vi "get_instrument_ID.vi"(8 "error in (no error)":errorcluster, 10 "ID Command":string="*IDN?\n", 11 "Function Generator in":refnum<class "Function Generator.lvclass">) -> (0 "error out":errorcluster, 2 "Instrument ID":string, 3 "Function Generator out":refnum<class "Function Generator.lvclass">)   [LabVIEW 2020, in "Function Generator.lvclass"]
uses:
  Function Generator.lvclass
  Function Generator.lvclass/Function Generator.ctl
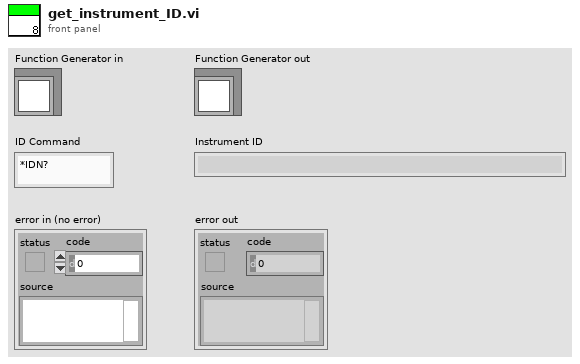
[diagram p1: front panel]
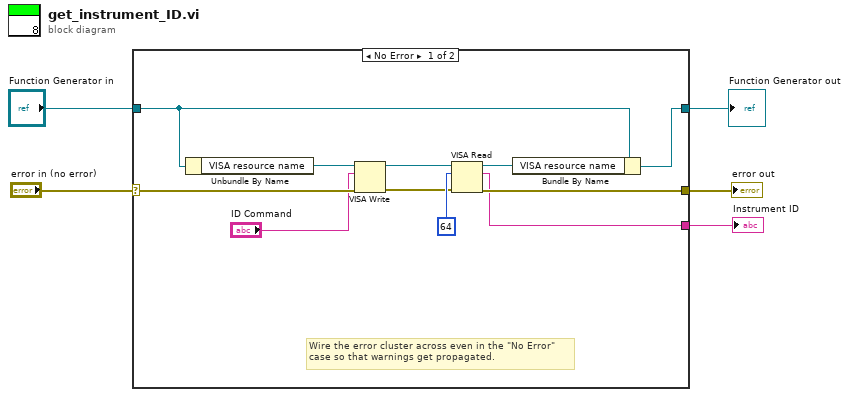
[diagram p0: block diagram]
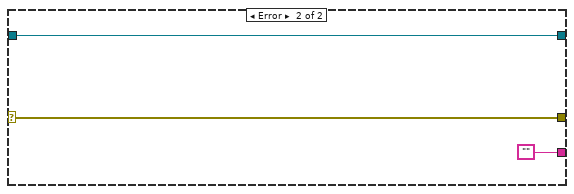
[diagram p2: hidden frame]
diagram:
  n1 = case shown="No Error" "error in (no error)" {
    selector: "error in (no error)" -> [w11 w19]
    tunnel: [w10 w19] -> w5
    tunnel: [w12 w18] -> w3
    tunnel: "Function Generator in" -> [w13 w18]
    tunnel: [w9 ""] -> w1
    frame No Error {
      # "Wire the error cluster across even in the \"No Error\"\ncase so that warnings get propagated."
      n2 = Unbundle By Name(w13) -> ("VISA resource name"=w16:refnum<visa-resource-name>)
      n3 = VISA Write(VISA resource name=w16, write buffer="ID Command", error in (no error)=w11) -> (VISA resource name out=w8:refnum<visa-resource-name>, error out=w7:errorcluster)  [unwired: 1 out]
      n4 = VISA Read(VISA resource name=w8, byte count=64, error in (no error)=w7) -> (VISA resource name out=w14:refnum<visa-resource-name>, read buffer=w9:string, error out=w10:errorcluster)  [unwired: 1 out]
      n5 = Bundle By Name(cluster=w13, "VISA resource name"=w14) -> (w12:refnum<class "Function Generator.lvclass">)
    }
    frame Error {
    }
  }
  "error out" <- w5
  "Function Generator out" <- w3
  "Instrument ID" <- w1
